vi "DeleteActionToRemainList.vi"(8 "error in (no error)":errorcluster, 9 "ManualFlg":bool, 10 "Remaining Action":refnum<vi>, 11 "MPC_VirbVision in":refnum<class "MPC_VirbVision.lvclass">) -> (0 "error out":errorcluster, 3 "MPC_VirbVision out":refnum<class "MPC_VirbVision.lvclass">)   [LabVIEW 2019, in "MPC_VirbVision.lvclass"]
uses:
  MPC_VirbVision.lvclass
  Main Class.lvclass
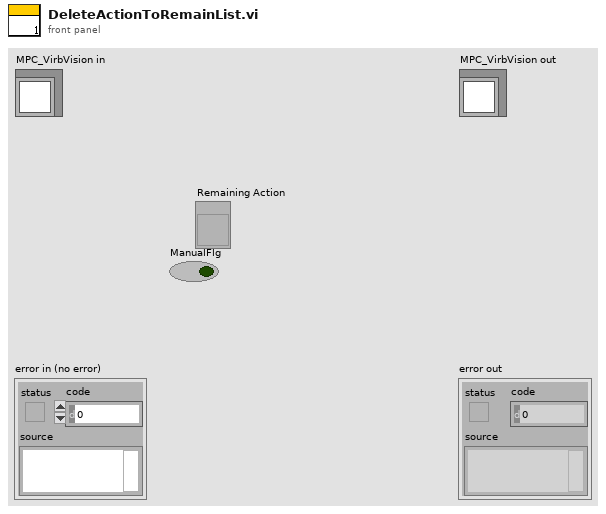
[diagram p1: front panel]
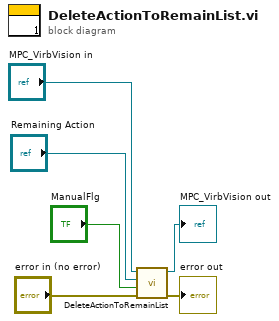
[diagram p0: block diagram]
diagram:
  n1 = call-parent "DeleteActionToRemainList.vi"("error in (no error)"="error in (no error)", "ManualFlg"="ManualFlg", "Remaining Action"="Remaining Action", "Main Class in"="MPC_VirbVision in") -> ("error out"=→"error out":errorcluster, "Main Class out"=→"MPC_VirbVision out":refnum<class "MPC_VirbVision.lvclass">)  [unwired: 6 in]
